vi "VI Snippet Export.vi"(8 "error in (no error)":errorcluster, 9 "Selected GObjects Only? (F)":bool, 10 "VI Refnum":refnum<vi>, 11 "VI Snippet Path (*.png)":path) -> (0 "error out":errorcluster)   [LabVIEW 2019, in "VI Snippet.lvlib"]
doc: "Exports a VI Snippet to the <b>VI Snippet Path (*.png)</b> specified and embeds the <b>VI Refnum</b> content. If <b>Selected GObjects Only?</b> is True, this exports the currently selected block diagram objects. Otherwise this exports the entire VI.\n\n<b>Errors:</b>\n<b>1026: \"VI reference is invalid\"</b> is raised if <b>VI Refnum</b> is \"Not a Refnum\".\n<b>1430: \"Empty path\"</b> is raised if the <b>VI Snippet Path (*.png)</b> is empty or not a path.\n\nCreated by: Ryan Pacini"
uses:
  VI Snippet.lvlib
  <vilib>/Utility/miscctls.llb/LVPositionTypeDef.ctl
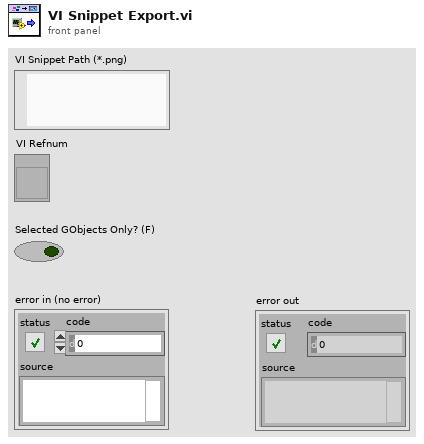
[diagram p1: front panel]
types:
  T1 = typedef "LVPositionTypeDef.ctl" = cluster{"Left":i32, "Top":i32}
  T2 = typedef "imagedata.ctl" = cluster{"image type":i32, "image depth":i32, "image":u8[], "mask":u8[], "colors":u32[], "Rectangle":cluster{"left":i16, "top":i16, "right":i16, "bottom":i16}}
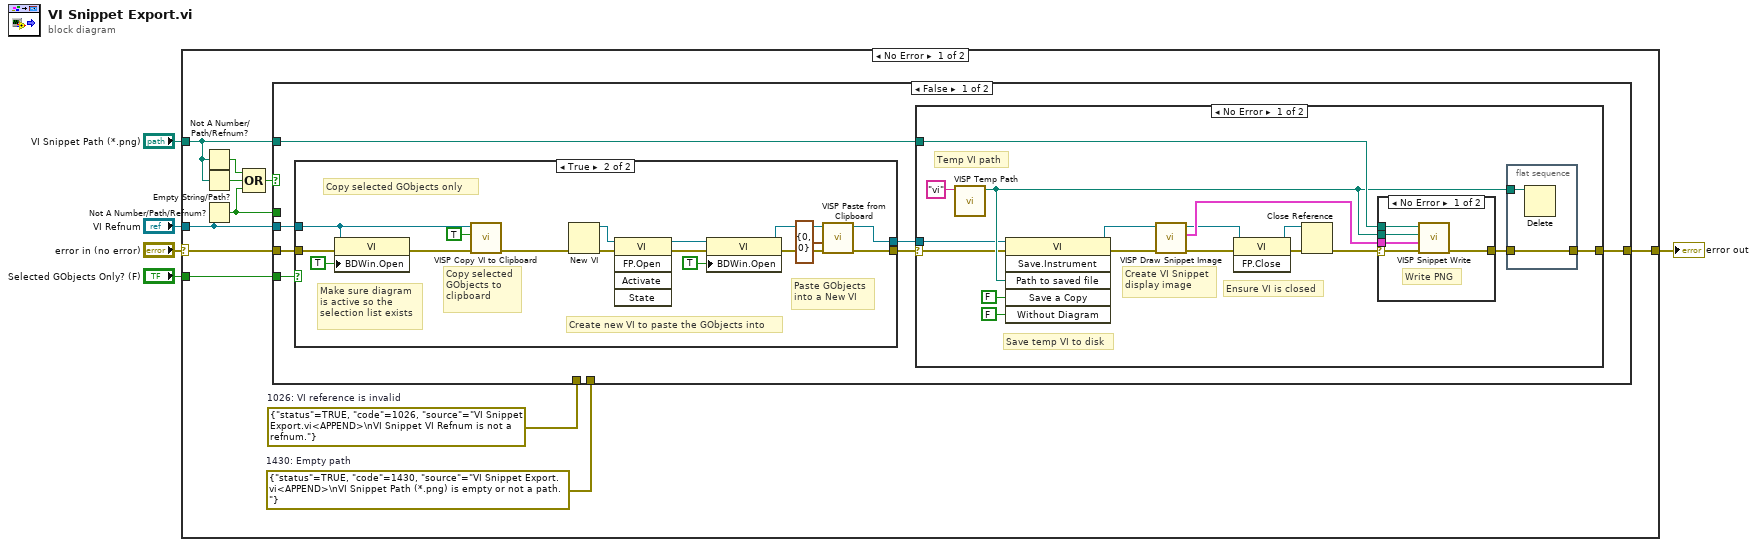
[diagram p0: block diagram]
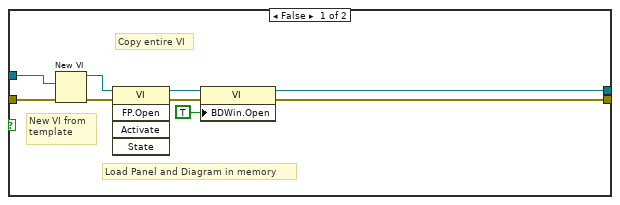
[diagram p4: hidden frame]
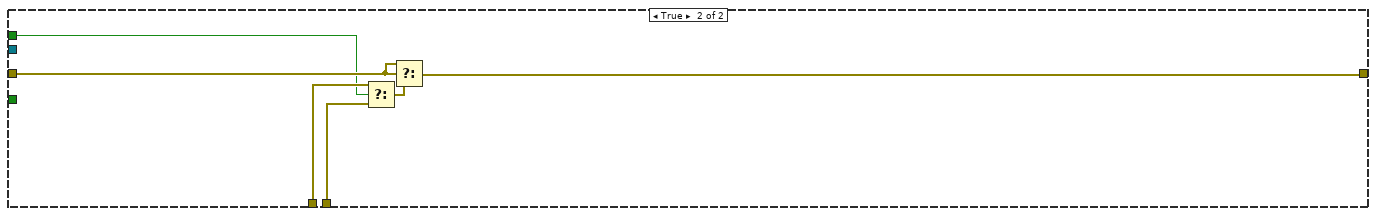
[diagram p5: hidden frame]
diagram:
  n1 = case shown="No Error" "error in (no error)" {
    selector: "error in (no error)" -> [w15 w81]
    tunnel: "VI Snippet Path (*.png)" -> [w12 _]
    tunnel: [w16 w81] -> w3
    tunnel: "VI Refnum" -> [w13 _]
    tunnel: "Selected GObjects Only? (F)" -> [w14 _]
    frame No Error {
      w6 = errorcluster {"status"=TRUE, "code"=1430, "source"="VI Snippet Export.vi<APPEND>\nVI Snippet Path (*.png) is empty or not a path."}  # 1430: Empty path
      w7 = errorcluster {"status"=TRUE, "code"=1026, "source"="VI Snippet Export.vi<APPEND>\nVI Snippet VI Refnum is not a refnum."}  # 1026: VI reference is invalid
      n2 = Not A Number/Path/Refnum?(number/path/refnum=w12) -> (NaN/Path/Refnum?=w10:bool)
      n3 = Empty String/Path?(string/path=w12) -> (empty?=w11:bool)
      n4 = Not A Number/Path/Refnum?(number/path/refnum=w13) -> (NaN/Path/Refnum?=w8:bool)
      n5 = Compound Arithmetic op=OR(w10, w11, w8) -> (w9:bool)
      n6 = case shown="False" w9 {
        tunnel: w12 -> [w23 _]
        tunnel: [w22 w79] -> w16
        tunnel: w15 -> [w21 w80]
        tunnel: w14 -> [w20 _]
        tunnel: w13 -> [w17 _]
        tunnel: w8 -> [_ w77]
        tunnel: w7 -> [_ w78]
        tunnel: w6 -> [_ w75]
        frame False {
          n7 = case shown="True" w20 {
            tunnel: w21 -> [w58 w74]
            tunnel: w17 -> [w57 w69]
            tunnel: [w54 w73] -> w19
            tunnel: [w50 w72] -> w18
            frame False {
              # "Load Panel and Diagram in memory"
              # "New VI from\ntemplate"
              # "Copy entire VI"
              n8 = New VI(8:w58, 10:w57) -> (0:w56:errorcluster, 3:w51:refnum<vi>)  [unwired: 5 in]
              n9 = invoke class="VI" method="FP.Open"(reference=w51, error in=w56) -> (reference out=w53:refnum<vi>, error out=w55:errorcluster)  [unwired: 3 in, 3 out]
              n10 = property class="VI"(reference=w53, error in=w55, "BDWin.Open"=TRUE ("Block Diagram Window:Open")) -> (reference out=w50:refnum<vi>, error out=w54:errorcluster)
            }
            frame True {
              # "Make sure diagram\nis active so the\nselection list exists"
              # "Create new VI to paste the GObjects into"
              # "Paste GObjects\ninto a New VI"
              # "Copy selected\nGObjects to\nclipboard"
              # "Copy selected GObjects only"
              n11 = property class="VI"(reference=w69, error in=w74, "BDWin.Open"=TRUE ("Block Diagram Window:Open")) -> (error out=w70:errorcluster)  [unwired: 1 out]
              n12 = call "VISP Copy VI to Clipboard.vi"("error in (no error)"=w70, "Selected GObjects Only? (F)"=TRUE, "VI Refnum in"=w69) -> ("error out"=w62:errorcluster)  [unwired: 7 in, 1 out]
              n13 = New VI(8:w62) -> (0:w67:errorcluster, 3:w66:refnum<vi>)  [unwired: 6 in]
              n14 = invoke class="VI" method="FP.Open"(reference=w66, error in=w67) -> (reference out=w65:refnum<vi>, error out=w64:errorcluster)  [unwired: 3 in, 3 out]
              n15 = property class="VI"(reference=w65, error in=w64, "BDWin.Open"=TRUE ("Block Diagram Window:Open")) -> (reference out=w60:refnum<vi>, error out=w61:errorcluster)
              n16 = call "VISP Paste from Clipboard.vi"("error in (no error)"=w61, "Drop Position (0, 0)"=T1 {"Left"=0, "Top"=0}, "VI Refnum in"=w60) -> ("error out"=w73:errorcluster, "VI Refnum out"=w72:refnum<vi>)  [unwired: 7 in]
            }
          }
          n17 = case shown="No Error" w19 {
            selector: w19 -> [w25 w49]
            tunnel: [w31 w49] -> w22
            tunnel: w23 -> [w40 _]
            tunnel: w18 -> [w24 _]
            frame No Error {
              # "Temp VI path"
              # "Create VI Snippet\ndisplay image"
              # "Ensure VI is closed"
              # "Save temp VI to disk"
              n18 = call "VISP Temp Path.vi"("Extension (\"vi\")"="vi" ("Extension (\"vi\")")) -> ("Path (*.png)"=w32:path)  [unwired: 10 in]
              n19 = invoke class="VI" method="Save.Instrument"(reference=w24, error in=w25, "Path to saved file"=w32, "Save a Copy"=FALSE, "Without Diagram"=FALSE) -> (reference out=w28:refnum<vi>, error out=w29:errorcluster)  [unwired: 1 in, 4 out]
              n20 = call "VISP Draw Snippet Image.vi"("error in (no error)"=w29, "VI Refnum in"=w28) -> ("error out"=w27:errorcluster, "Image Data"=w39:T2, "dup VI Refnum"=w26:refnum<vi>)  [unwired: 7 in]
              n21 = invoke class="VI" method="FP.Close"(reference=w26, error in=w27) -> (reference out=w35:refnum<vi>, error out=w36:errorcluster)  [unwired: 1 in, 1 out]
              n22 = Close Reference(reference=w35, error in (no error)=w36) -> (error out=w33:errorcluster)
              n23 = case shown="No Error" w33 {
                selector: w33 -> [w44 w46]
                tunnel: w40 -> [w45 _]
                tunnel: w39 -> [w41 _]
                tunnel: w32 -> [w42 _]
                tunnel: [w43 w46] -> w30
                frame No Error {
                  # "Write PNG"
                  n24 = call "VISP Snippet Write.vi"("error in (no error)"=w44, "Image Data in"=w41, "VI Path (*.vi)"=w42, "VI Snippet Path (*.png)"=w45) -> ("error out"=w43:errorcluster)  [unwired: 7 in]
                }
                frame Error {
                }
              }
              n25 = flat-sequence {
                tunnel: w32 -> [w48]
                tunnel: [w47] -> w31
                tunnel: w30 -> [w47]
                frame #0 {
                  n26 = Delete(path (use dialog)=w48) -> ()  [unwired: 4 in, 3 out]
                }
              }
            }
            frame Error {
            }
          }
        }
        frame True {
          n27 = Select(t=w78, s=w77, f=w75) -> (s? t:f=w76:errorcluster)
          n28 = Select(t=w80, s=w80, f=w76) -> (s? t:f=w79:errorcluster)
        }
      }
    }
    frame Error {
    }
  }
  "error out" <- w3
